vi "Reset RX FIFO.vi"(0 "Refnum in":refnum<k20>, 5 "Port":T1 items=["Port 0", "Port 1", "Port 2", "Port 3"], 7 "stream index":i32, 11 "error in":errorcluster) -> (4 "Refnum out":refnum<k20>, 15 "error out":errorcluster)   [LabVIEW 2016, in "Aurora Stream (NI 6592R) (Host).lvlib"]
doc: "Requests the stream to clear, which commands it to \"Idle.\" When the stream goes idle, the FIFO connected to <b>Port</b> is stopped to clear it of samples.\n\n<B>Input Parameters</B>\n\n<B>Refnum in</B> Receives a reference to the FPGA from the previous VI.\n\n<B>Port</B> Specifies the physical port whose stream will be cleared.\n\n<B>error in</B> describes error conditions that occur before this node runs. This input provides standard error in functionality.\n\n<B>Output Parameters</B>\n\n<B>Refnum out</B> passes a reference to the FPGA to the next VI.\n\n<B>error out</B> contains error information. This output provides standard error out functionality."
uses:
  Aurora Stream (NI 6592R) (Host).lvlib
  Port.ctl
  Base Bitfile Reference.ctl
  <vilib>/Utility/error.llb/Error Cluster From Error Code.vi
  <vilib>/rvi/interface/nirviMethod/nirviMethod.xnode
  <instrlib>/_niInstr/Streaming/v1/Host/niInstr Streaming v1 Host.lvlib
  <vilib>/FPGAPlugInAG/Dynamic/niLvFpga_StopFifo_Dynamic.vi
  <vilib>/rvi/errors/niLvFpgaMergeErrorWithErrorCode.vi
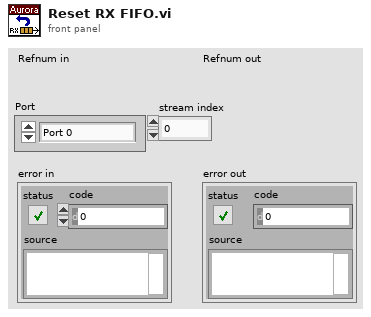
[diagram p1: front panel]
types:
  T1 = typedef "Aurora Stream (NI 6592R) (Host).lvlib/Port.ctl" = i32
  T2 = typedef "Aurora Stream (NI 6592R) (Host).lvlib/Base Bitfile Reference.ctl" = refnum<k20>
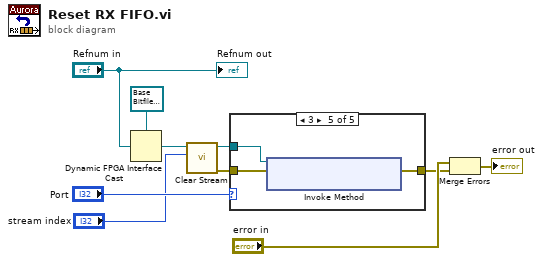
[diagram p0: block diagram]
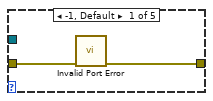
[diagram p2: hidden frame]
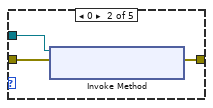
[diagram p3: hidden frame]
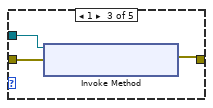
[diagram p4: hidden frame]
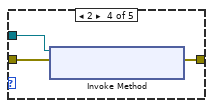
[diagram p5: hidden frame]
diagram:
  n1 = Dynamic FPGA Interface Cast(Session In=T2 refnum ("Aurora Sample Project"), Type="Refnum in") -> (Session Out=w3:T2)
  n2 = call <instrlib>:"Clear Stream.vi"("stream index"="stream index", "refnum in"=w3) -> ("error out"=w6:errorcluster, "refnum out"=w7:T2)  [unwired: 8 in]
  n3 = case shown="3" "Port" {
    tunnel: [w12 w15 w16 w21 w22] -> w8
    tunnel: w7 -> [_ w14 w17 w20 w23]
    tunnel: w6 -> [w11 w13 w18 w19 w24]
    frame -1, Default {
      n4 = call "Invalid Port Error.vi"("error in"=w11) -> ("error out"=w12:errorcluster)  [unwired: 14 in]
    }
    frame 0 {
      n5 = xnode "Invoke Method"("FPGA VI Reference In"=w14, "error in"=w13) -> ("error out"=w15:errorcluster)  [unwired: 1 out]
    }
    frame 1 {
      n6 = xnode "Invoke Method"("FPGA VI Reference In"=w17, "error in"=w18) -> ("error out"=w16:errorcluster)  [unwired: 1 out]
    }
    frame 2 {
      n7 = xnode "Invoke Method"("FPGA VI Reference In"=w20, "error in"=w19) -> ("error out"=w21:errorcluster)  [unwired: 1 out]
    }
    frame 3 {
      n8 = xnode "Invoke Method"("FPGA VI Reference In"=w23, "error in"=w24) -> ("error out"=w22:errorcluster)  [unwired: 1 out]
    }
  }
  n9 = Merge Errors("error in", w8) -> (→"error out":errorcluster)
  "Refnum out" <- "Refnum in"
